vi "User Defined Collections.vi"(8 "error in (no error)":errorcluster, 11 "Node Ptr":T1 format="%.0x") -> (0 "error out":errorcluster)   [LabVIEW 2015, in "Diagnostics Addon System Explorer.lvlib"]
uses:
  Diagnostics Addon System Explorer.lvlib
  <vilib>/NI Veristand/Custom Device API/Custom Device Item Ref.ctl
  Shared/SubVIs/Constants.vi
  <vilib>/NI Veristand/Custom Device Tools/Custom Device Utility Library/NI VeriStand - Search for All Items by GUID.vi
  <vilib>/NI Veristand/Custom Device API/Custom Device API.lvlib
  <vilib>/NI Veristand/Custom Device Tools/Custom Device Utility Library/Custom Device Utility Library.lvlib
  Shared/Diagnostics Addon Shared.lvlib
panel:
  in  "SHDocVw.IWebBrowser":refnum<k7>(container)
  in  "Collection":i32(listbox) caption="User Defined Messages"
  in  "Description":string
  in  "Name Control":string caption="Name"
  in  "Header":cluster{"Section Name":string}={"Section Name"="Custom Device Item Settings"}
  out "Name":string
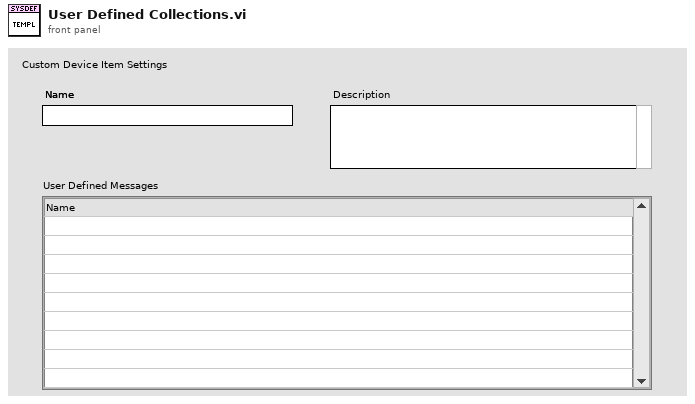
[diagram p1: front panel]
types:
  T1 = typedef "Custom Device API.lvlib/Custom Device Item Ref.ctl" = u64
  T2 = typedef "Custom Device API.lvlib/Custom Device Item Info.ctl" = cluster{"Name":string, "Is Channel":bool, "GUID":string, "Is Waveform":bool}
  T3 = typedef "Custom Device API.lvlib/Custom Device Commands.ctl" = enum16{"Default", "Item renamed", "Shutdown", "Dynamic button pressed"}
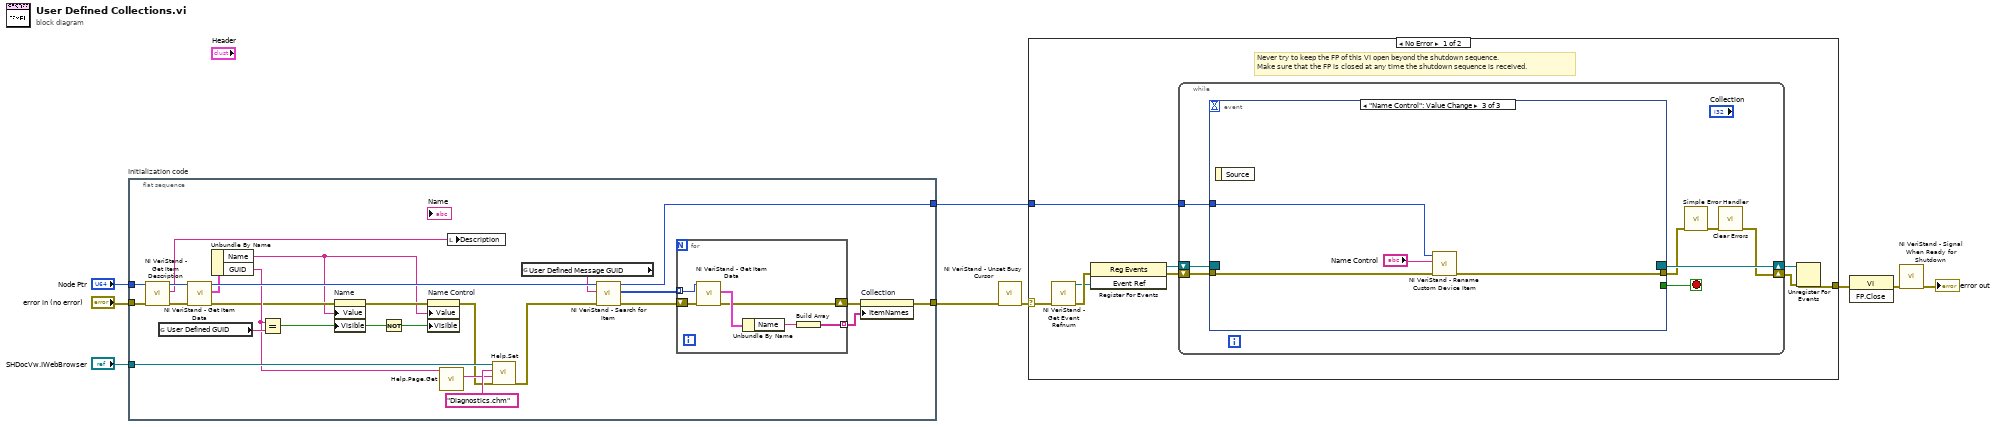
[diagram p0: block diagram]
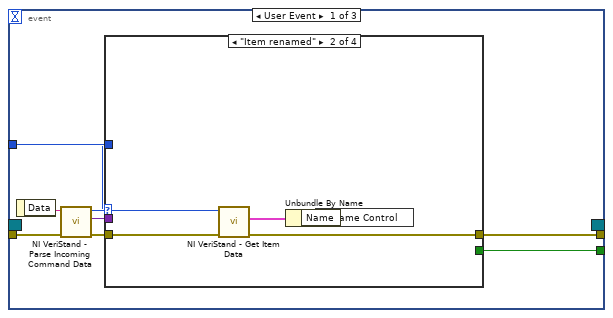
[diagram p2: hidden frame]
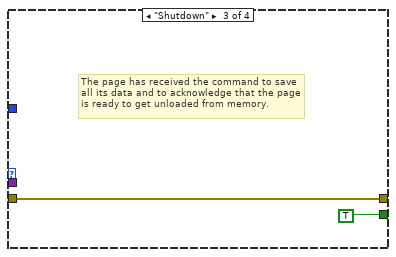
[diagram p4: hidden frame]
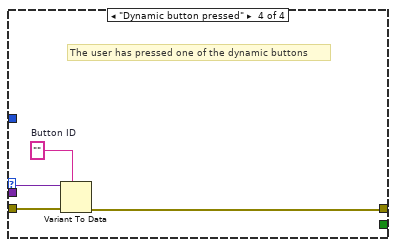
[diagram p5: hidden frame]
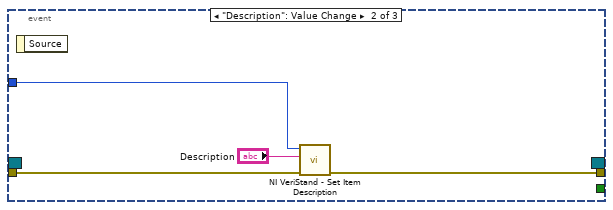
[diagram p6: hidden frame]
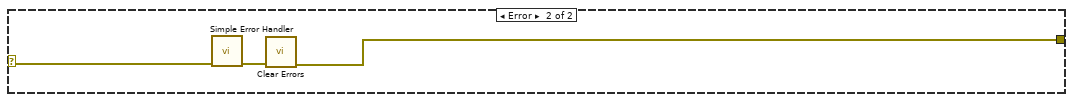
[diagram p7: hidden frame]
diagram:
  n1 = flat-sequence "Initialization code" {
    tunnel: "error in (no error)" -> [w20]
    tunnel: [w24] -> w6
    tunnel: [w26] -> w3
    tunnel: "Node Ptr" -> [w29]
    tunnel: "SHDocVw.IWebBrowser" -> [w21]
    frame #0 {
      n2 = call <vilib>:"NI VeriStand - Get Item Description.vi"("error in (no error)"=w20, "Item Ref in"=w29) -> ("error out"=w32:errorcluster, "Description"=w33:string, "Item Ref out"=w34:T1)  [unwired: 7 out]
      n3 = global read "Constants.vi" "User Defined GUID"() -> (w16:string)
      n4 = call <vilib>:"NI VeriStand - Get Item Data.vi"("error in (no error)"=w32, "Item Ref in"=w34) -> ("error out"=w14:errorcluster, "Item Info"=w31:T2, "Item Ref out"=w35:T1)  [unwired: 7 out]
      n5 = Unbundle By Name(w31) -> ("Name"=w12:string, "GUID"=w15:string)
      n6 = Equal?(x=w15, y=w16) -> (x = y?=w10:bool)
      n7 = property on="Name" class="Str"(error in=w14, "Value"=w12, "Visible"=w10) -> (error out=w13:errorcluster)  [unwired: 1 in, 1 out]
      n8 = Not(x=w10) -> (.not. x?=w11:bool)
      n9 = property on="Name Control" class="Str"(error in=w13, "Value"=w12, "Visible"=w11) -> (error out=w17:errorcluster)  [unwired: 1 in, 1 out]
      n10 = call "Help.Page.Get.vi"("GUID"=w15) -> ("HTML File"=w22:string)  [unwired: 10 in]
      n11 = local write "Description"(w33) -> ()
      n12 = call "Help.Set.vi"("error in (no error)"=w17, "HTML File"=w22, "Main CHM File"="Diagnostics.chm", "SHDocVw.IWebBrowser2"=w21) -> ("error out"=w23:errorcluster)  [unwired: 7 in]
      n13 = global read "Constants.vi" "User Defined Message GUID"() -> (w18:string)
      n14 = call-poly <vilib>:"NI VeriStand - Search for Item.vi"("error in"=w23, "Item GUID"=w18, "Section Ref in"=w35) -> ("error out"=w28:errorcluster, "Item Refs"=w27:T1[], "Section Ref out"=w26:T1)  [unwired: 5 in, 1 out]
      n15 = for {
        shift-right: [w38] -> w25
        shift-left: w28 -> [w41]
        tunnel: w27 -> [w40] mode=indexing
        tunnel: [w36] -> w19 mode=indexing
        n16 = call <vilib>:"NI VeriStand - Get Item Data.vi"("error in (no error)"=w41, "Item Ref in"=w40) -> ("error out"=w38:errorcluster, "Item Info"=w39:T2)  [unwired: 8 out]
        n17 = Unbundle By Name(w39) -> ("Name"=w37:string)
        n18 = Build Array(w37) -> (w36:string[])
      }
      n19 = property on="Collection" class="MCListbox (strict)"(error in=w25, "ItemNames"=w19) -> (error out=w24:errorcluster)  [unwired: 1 in, 1 out]
    }
  }
  n20 = call <vilib>:"NI VeriStand - Unset Busy Cursor.vi"("error in (no error)"=w6) -> ("error out"=w5:errorcluster)  [unwired: 10 out]
  n21 = case shown="No Error" w5 {
    selector: w5 -> [w42 w89]
    tunnel: [w47 w87] -> w9
    tunnel: w3 -> [w43 _]
    frame No Error {
      # "Never try to keep the FP of this VI open beyond the shutdown sequence.\nMake sure that the FP is closed at any time the shutdown sequence is received."
      n22 = call <vilib>:"NI VeriStand - Get Event Refnum.vi"("error in (no error)"=w42) -> ("error out"=w50:errorcluster, "Event Ref"=w46:refnum<user-event>)  [unwired: 9 out]
      n23 = register-events(error in=w50, w46) -> (reference out=w44:refnum<event-registration>, error out=w45:errorcluster)  [unwired: 1 in]
      n24 = while {
        tunnel: w43 -> [w54]
        shift-right: [w51] -> w48
        shift-left: w45 -> [w57]
        shift-right: [w58] -> w49
        shift-left: w44 -> [w56]
        stop <- w55 stop-if-true
        n25 = event shown="[2] \"Name Control\": Value Change" {
          selector: w56 -> [_ _ _]
          dyn-events: [_ _ _] -> w58
          timeout: _ -> [_ _ _]
          tunnel: w57 -> [w66 w81 w85]
          tunnel: [w62 _ _] -> w55
          tunnel: [w61 w80 w84] -> w53
          tunnel: w54 -> [w60 w82 w86]
          event User Event {
            n26 = event-data() -> ("Data"=w65:string)  [unwired: 1 out]
            n27 = call <vilib>:"NI VeriStand - Parse Incoming Command Data.vi"("error in (no error)"=w66, "Incoming data"=w65) -> ("error out"=w64:errorcluster, "Outgoing data"=w59:variant, "Action"=w63:T3)  [unwired: 7 out]
            n28 = case shown="\"Item renamed\"" w63 {
              tunnel: w64 -> [w67 w72 w73 w78]
              tunnel: [_ _ TRUE _] -> w62
              tunnel: [w67 w69 w73 w75] -> w61
              tunnel: w60 -> [_ w71 _ _]
              tunnel: w59 -> [_ _ _ w77]
              frame "Default", Default {
              }
              frame "Item renamed" {
                n29 = call <vilib>:"NI VeriStand - Get Item Data.vi"("error in (no error)"=w72, "Item Ref in"=w71) -> ("error out"=w69:errorcluster, "Item Info"=w70:T2)  [unwired: 8 out]
                n30 = Unbundle By Name(w70) -> ("Name"=w68:string)
                n31 = local write "Name Control"(w68) -> ()
              }
              frame "Shutdown" {
                # "The page has received the command to save all its data and to acknowledge that the page is ready to get unloaded from memory."
              }
              frame "Dynamic button pressed" {
                w76 = ""  # Button ID
                # "The user has pressed one of the dynamic buttons"
                n32 = Variant To Data(error in=w78, type=w76, Variant=w77) -> (error out=w75:errorcluster)  [unwired: 1 out]
              }
            }
          }
          event "Description": Value Change {
            n33 = event-data() -> ()  [unwired: 2 out]
            n34 = call <vilib>:"NI VeriStand - Set Item Description.vi"("error in (no error)"=w81, "Description"="Description", "Item Ref in"=w82) -> ("error out"=w80:errorcluster)  [unwired: 8 out]
          }
          event "Name Control": Value Change {
            n35 = event-data() -> ()  [unwired: 2 out]
            n36 = call <vilib>:"NI VeriStand - Rename Custom Device Item.vi"("error in (no error)"=w85, "New Name"="Name Control", "Item Ref in"=w86) -> ("error out"=w84:errorcluster)  [unwired: 6 in, 2 out]
          }
        }
        n37 = call <vilib>:"Simple Error Handler.vi"("error in (no error)"=w53) -> ("error out"=w52:errorcluster)  [unwired: 1 in, 7 out]
        n38 = call <vilib>:"Clear Errors.vi"("error in (no error)"=w52) -> ("error out"=w51:errorcluster)  [unwired: 1 in, 5 out]
      }
      n39 = Unregister For Events(event registration refnum=w49, error in=w48) -> (error out=w47:errorcluster)
    }
    frame Error {
      n40 = call <vilib>:"Simple Error Handler.vi"("error in (no error)"=w89) -> ("error out"=w88:errorcluster)  [unwired: 1 in, 7 out]
      n41 = call <vilib>:"Clear Errors.vi"("error in (no error)"=w88) -> ("error out"=w87:errorcluster)  [unwired: 1 in, 5 out]
    }
  }
  n42 = invoke class="VI" method="FP.Close"(error in=w9) -> (error out=w8:errorcluster)  [unwired: 2 in, 2 out]
  n43 = call <vilib>:"NI VeriStand - Signal When Ready for Shutdown.vi"("error in (no error)"=w8) -> ("error out"=→"error out":errorcluster)  [unwired: 10 out]
